vi "Frisbee Vision Cluster Sorter.vi"(0 "input cluster":T1, 1 "input cluster 2":T1, 5 "input cluster 3":T1, 6 "input cluster 4":T1) -> (7 "Chosen Particle Info":T1)   [LabVIEW 2012]
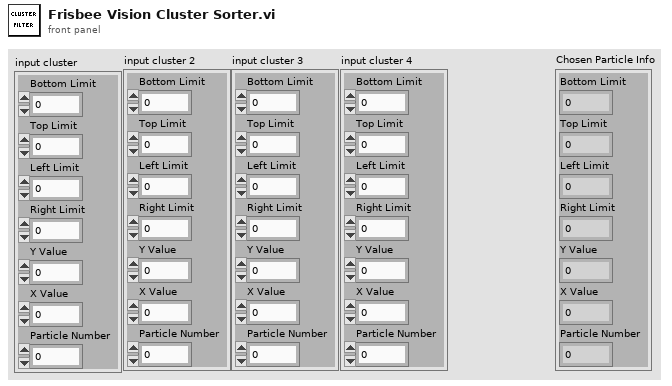
[diagram p1: front panel]
types:
  T1 = cluster{"Bottom Limit":i32, "Top Limit":i32, "Left Limit":i32, "Right Limit":i32, "Y Value":i32, "X Value":i32, "Particle Number":i32}
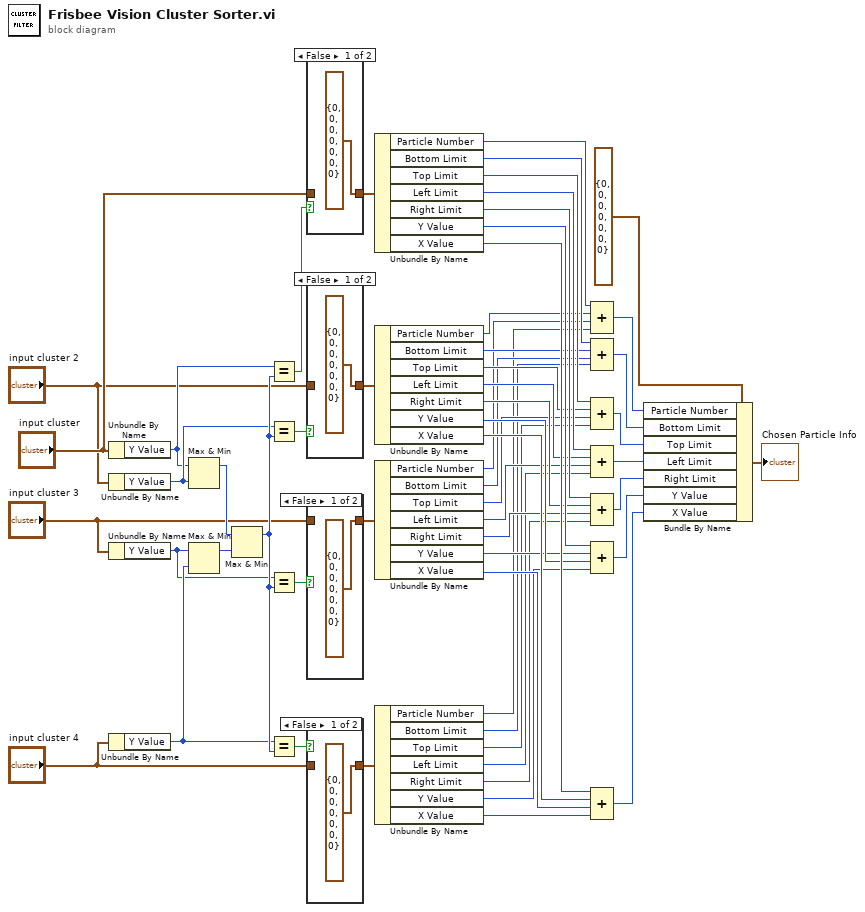
[diagram p0: block diagram]
diagram:
  n1 = Unbundle By Name("input cluster") -> ("Y Value"=w50:i32)
  n2 = Unbundle By Name("input cluster 2") -> ("Y Value"=w51:i32)
  n3 = Unbundle By Name("input cluster 3") -> ("Y Value"=w52:i32)
  n4 = Unbundle By Name("input cluster 4") -> ("Y Value"=w53:i32)
  n5 = Max & Min(x=w50, y=w51) -> (max(x,y)=w56:i32)  [unwired: 1 out]
  n6 = Max & Min(x=w52, y=w53) -> (max(x,y)=w55:i32)  [unwired: 1 out]
  n7 = Max & Min(x=w56, y=w55) -> (max(x,y)=w54:i32)  [unwired: 1 out]
  n8 = Equal?(x=w50, y=w54) -> (x = y?=w49:bool)
  n9 = Equal?(x=w51, y=w54) -> (x = y?=w47:bool)
  n10 = Equal?(x=w52, y=w54) -> (x = y?=w45:bool)
  n11 = Equal?(x=w53, y=w54) -> (x = y?=w43:bool)
  n12 = case shown="False" w49 {
    tunnel: [T1 {"Bottom Limit"=0, "Top Limit"=0, "Left Limit"=0, "Right Limit"=0, "Y Value"=0, "X Value"=0, "Particle Number"=0} ("input cluster") w58] -> w41
    tunnel: "input cluster" -> [_ w58]
    frame False {
    }
    frame True {
    }
  }
  n13 = case shown="False" w47 {
    tunnel: [T1 {"Bottom Limit"=0, "Top Limit"=0, "Left Limit"=0, "Right Limit"=0, "Y Value"=0, "X Value"=0, "Particle Number"=0} ("input cluster") w60] -> w40
    tunnel: "input cluster 2" -> [_ w60]
    frame False {
    }
    frame True {
    }
  }
  n14 = case shown="False" w45 {
    tunnel: [T1 {"Bottom Limit"=0, "Top Limit"=0, "Left Limit"=0, "Right Limit"=0, "Y Value"=0, "X Value"=0, "Particle Number"=0} ("input cluster") w62] -> w39
    tunnel: "input cluster 3" -> [_ w62]
    frame False {
    }
    frame True {
    }
  }
  n15 = case shown="False" w43 {
    tunnel: [T1 {"Bottom Limit"=0, "Top Limit"=0, "Left Limit"=0, "Right Limit"=0, "Y Value"=0, "X Value"=0, "Particle Number"=0} ("input cluster") w64] -> w38
    tunnel: "input cluster 4" -> [_ w64]
    frame False {
    }
    frame True {
    }
  }
  n16 = Unbundle By Name(w41) -> ("Particle Number"=w37:i32, "Bottom Limit"=w36:i32, "Top Limit"=w35:i32, "Left Limit"=w34:i32, "Right Limit"=w33:i32, "Y Value"=w32:i32, "X Value"=w31:i32)
  n17 = Unbundle By Name(w40) -> ("Particle Number"=w30:i32, "Bottom Limit"=w29:i32, "Top Limit"=w28:i32, "Left Limit"=w27:i32, "Right Limit"=w26:i32, "Y Value"=w25:i32, "X Value"=w24:i32)
  n18 = Unbundle By Name(w39) -> ("Particle Number"=w23:i32, "Bottom Limit"=w22:i32, "Top Limit"=w21:i32, "Left Limit"=w20:i32, "Right Limit"=w19:i32, "Y Value"=w18:i32, "X Value"=w17:i32)
  n19 = Unbundle By Name(w38) -> ("Particle Number"=w10:i32, "Bottom Limit"=w11:i32, "Top Limit"=w12:i32, "Left Limit"=w13:i32, "Right Limit"=w14:i32, "Y Value"=w15:i32, "X Value"=w16:i32)
  n20 = Compound Arithmetic op=ADD(w37, w30, w23, w10) -> (w8:i32)
  n21 = Compound Arithmetic op=ADD(w36, w29, w22, w11) -> (w7:i32)
  n22 = Compound Arithmetic op=ADD(w35, w28, w21, w12) -> (w6:i32)
  n23 = Compound Arithmetic op=ADD(w34, w27, w20, w13) -> (w5:i32)
  n24 = Compound Arithmetic op=ADD(w33, w26, w19, w14) -> (w4:i32)
  n25 = Compound Arithmetic op=ADD(w32, w18, w25, w15) -> (w3:i32)
  n26 = Compound Arithmetic op=ADD(w31, w24, w17, w16) -> (w2:i32)
  n27 = Bundle By Name(cluster=T1 {"Bottom Limit"=0, "Top Limit"=0, "Left Limit"=0, "Right Limit"=0, "Y Value"=0, "X Value"=0, "Particle Number"=0} ("input cluster"), "Particle Number"=w8, "Bottom Limit"=w7, "Top Limit"=w6, "Left Limit"=w5, "Right Limit"=w4, "Y Value"=w3, "X Value"=w2) -> (→"Chosen Particle Info":T1)
